vi "code4.vi"() -> ()   [LabVIEW 2019]
panel:
  in  "Stop":bool
  in  "A":dbl
  in  "B":dbl(knob) scale=0.0..10.0
  out "Waveform Chart":dbl(graph)
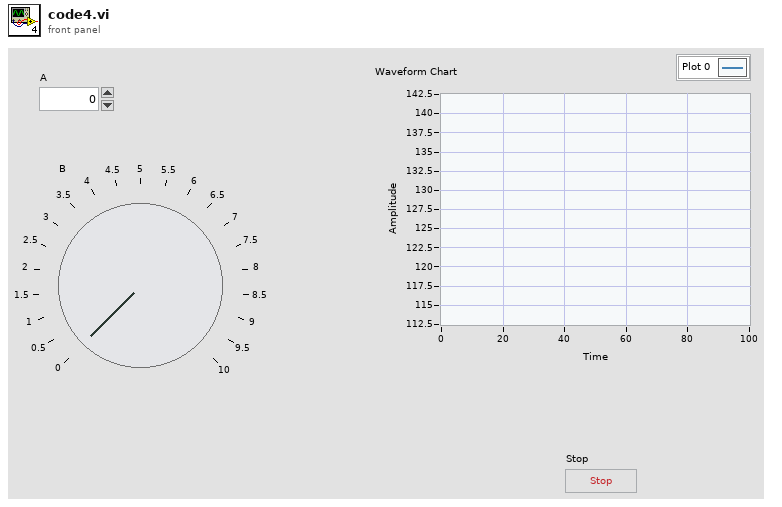
[diagram p1: front panel]
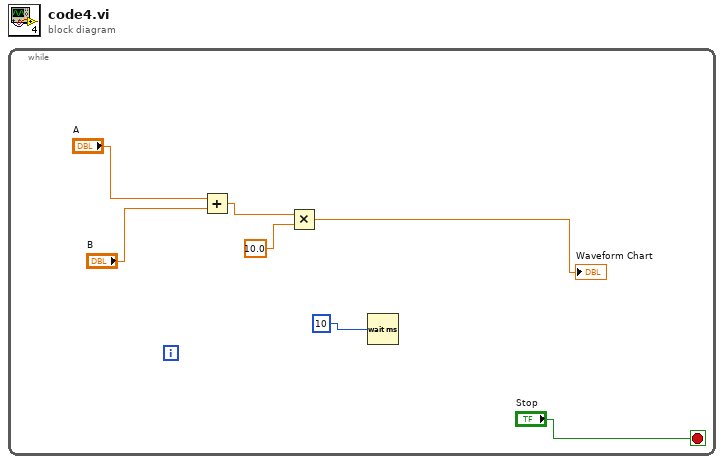
[diagram p0: block diagram]
diagram:
  n1 = while {
    stop <- "Stop" stop-if-true
    n2 = Add(x="A", y="B") -> (x+y=w5:dbl)
    n3 = Multiply(x=w5, y=10.0) -> (x*y=→"Waveform Chart":dbl)
    n4 = Wait (ms)(milliseconds to wait=10) -> ()  [unwired: 1 out]
  }
